vi "GOOP_GetGDSConfigFolder.vi"() -> (0 "GDSFolderPath":path)   [LabVIEW 2016]
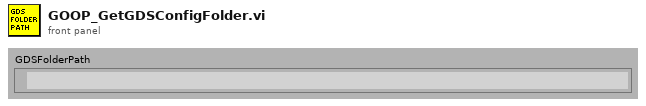
[diagram p1: front panel]
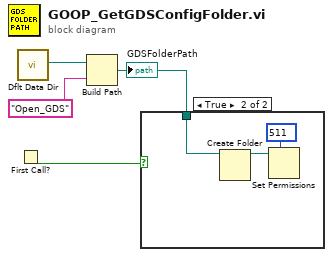
[diagram p0: block diagram]
diagram:
  n1 = First Call?() -> (First Call?: T/F=w2:bool)
  n2 = call <vilib>:"Dflt Data Dir.vi"() -> ("App:Default Data Directory"=w4:path)
  n3 = Build Path(base path=w4, name or relative path="Open_GDS") -> (appended path=w1:path)
  "GDSFolderPath" <- w1
  n4 = case shown="True" w2 {
    tunnel: w1 -> [_ w7]
    frame False {
    }
    frame True {
      n5 = Create Folder(path (use dialog)=w7) -> (created path=w5:path)  [unwired: 2 in, 2 out]
      n6 = Set Permissions(7:i16 511 ("permissions"), 11:w5) -> ()  [unwired: 3 in, 2 out]
    }
  }
